vi "Delete Array DVR.vi"(8 "error in (no error)":errorcluster, 11 "Array DVR in":refnum<data-value>) -> (0 "error out":errorcluster, 3 "Array out":refnum<class "Array.lvclass">)   [LabVIEW 2012, in "MDSplus.lvlib" / "Array.lvclass"]
uses:
  <vilib>/MDSplus/Classes/Data_Class/Array_Class/Array.lvclass
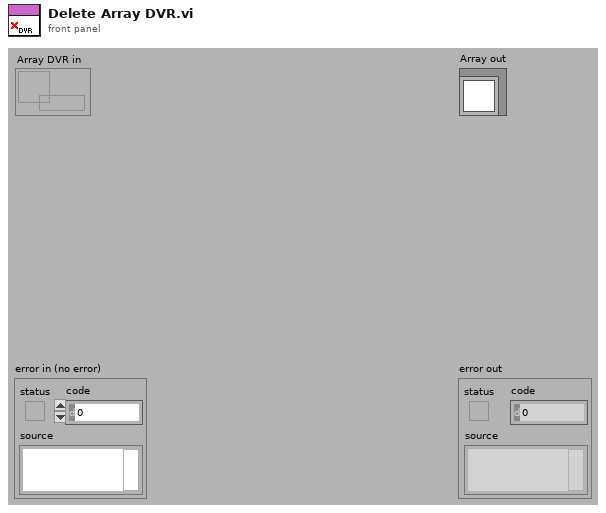
[diagram p1: front panel]
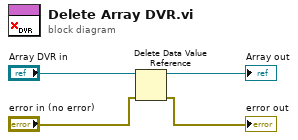
[diagram p0: block diagram]
diagram:
  n1 = Delete Data Value Reference(data value reference="Array DVR in", error in="error in (no error)") -> (data value=→"Array out":refnum<class "Array.lvclass">, error out=→"error out":errorcluster)
